vi "Fold remaining string.vi"(4 "index":i32, 5 "after match":string, 7 "before match":string) -> (3 "remaining":string)   [LabVIEW 2020, in "NI_WFCN.lvlib"]
doc: "If the previous string match succeeded, returns what was remaining after the match. Otherwise, returns the original (unmatched) string."
uses:
  <vilib>/net/WFCN/NI_WFCN.lvlib
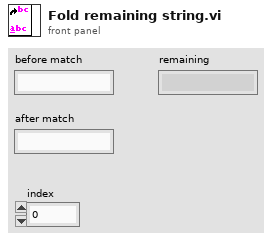
[diagram p1: front panel]
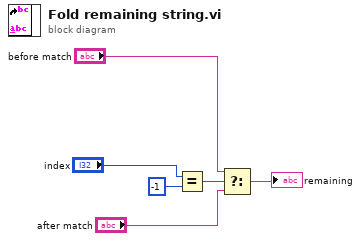
[diagram p0: block diagram]
diagram:
  n1 = Equal?(x="index", y=-1) -> (x = y?=w4:bool)
  n2 = Select(t="before match", s=w4, f="after match") -> (s? t:f=→"remaining":string)
